vi "Convert cxd file.vi"(8 "error in (no error)":errorcluster, 11 "TomoConversion in":refnum<class "TomoConversion.lvclass">) -> (0 "error out":errorcluster, 3 "TomoConversion out":refnum<class "TomoConversion.lvclass">)   [LabVIEW 2012, in "TomoConversion.lvclass"]
uses:
  TomoConversion.lvclass
  TomoConversion.lvclass/TomoConversion.ctl
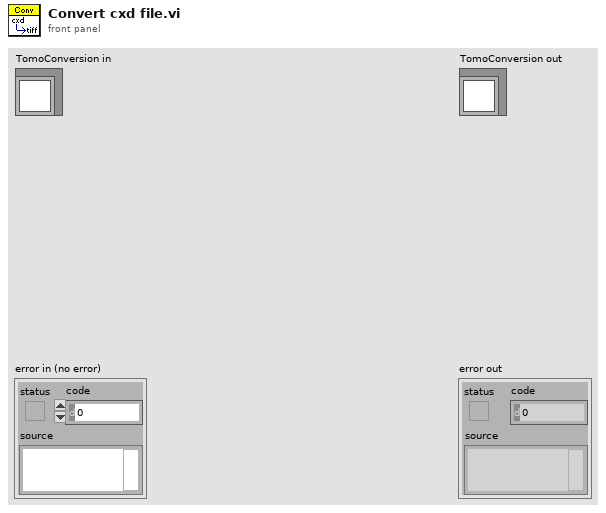
[diagram p1: front panel]
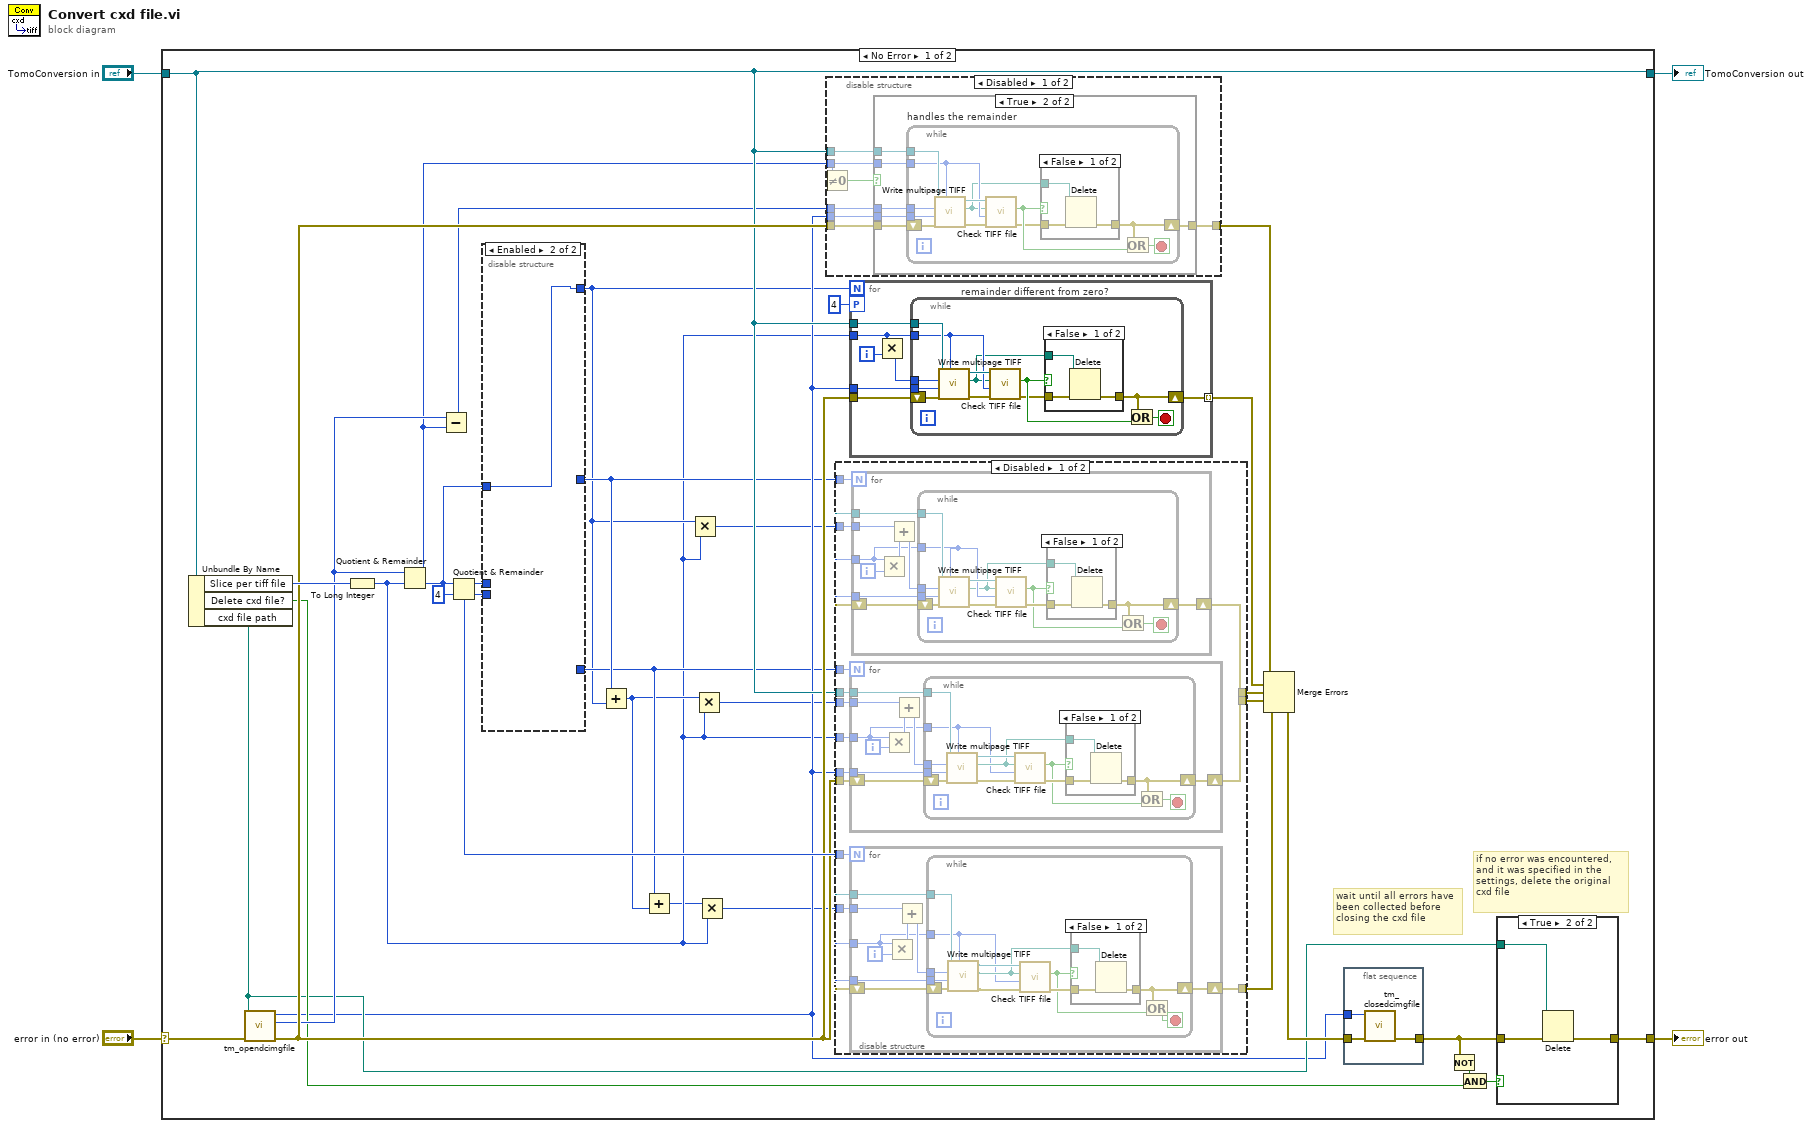
[diagram p0: block diagram]
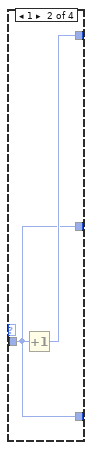
[diagram p3: hidden frame]
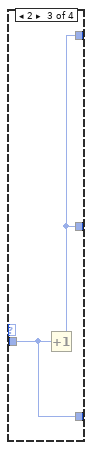
[diagram p4: hidden frame]
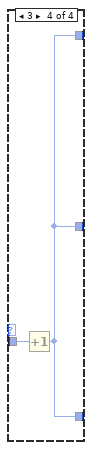
[diagram p5: hidden frame]
diagram:
  n1 = case shown="No Error" "error in (no error)" {
    selector: "error in (no error)" -> [w31 w201]
    tunnel: [w20 w201] -> w3
    tunnel: [w29 w200] -> w1
    tunnel: "TomoConversion in" -> [w29 w200]
    frame No Error {
      # "wait until all errors have\nbeen collected before\nclosing the cxd file"
      # "if no error was encountered, \nand it was specified in the \nsettings, delete the original\ncxd file"
      n2 = Unbundle By Name(w29) -> ("Slice per tiff file"=w38:u32, "Delete cxd file?"=w23:bool, "cxd file path"=w19:path)
      n3 = call <userlib>:"tm_opendcimgfile.vi"("error in (no error)"=w31, "Path"=w19) -> ("error out"=w30:errorcluster, "Total Frames"=w28:i32, "File Handle"=w17:u32)  [unwired: 7 in]
      n4 = To Long Integer(number=w38) -> (32bit integer=w9:i32)
      n5 = Quotient & Remainder(x=w28, y=w9) -> (x-y*floor(x/y)=w18:i32, floor(x/y)=w6:i32)
      n6 = Subtract(x=w28, y=w18) -> (x-y=w27:i32)
      n7 = Quotient & Remainder(x=w6, y=4) -> (x-y*floor(x/y)=w16:i32, floor(x/y)=w36:i32)
      n8 = disable-structure shown="Enabled" {
        disable-tunnel: w36 -> [w43 _]
        disable-tunnel: w16 -> [w42 _]
        disable-tunnel: [w41 _] -> w15
        disable-tunnel: [w40 _] -> w14
        disable-tunnel: [w39 w51] -> w13
        disable-tunnel: w6 -> [_ w51]
        frame Disabled {
          n9 = case shown="0, Default" w42 {
            tunnel: w43 -> [w44 w45 w48 w50]
            tunnel: [w44 w46 w47 w49] -> w39
            tunnel: [w44 w45 w47 w49] -> w41
            tunnel: [w44 w45 w48 w49] -> w40
            frame 0, Default {
            }
            frame 1 {
              n10 = Increment(x=w45) -> (x+1=w46:i32)
            }
            frame 2 {
              n11 = Increment(x=w48) -> (x+1=w47:i32)
            }
            frame 3 {
              n12 = Increment(x=w50) -> (x+1=w49:i32)
            }
          }
        }
        frame Enabled {
        }
      }
      n13 = Add(x=w15, y=w13) -> (x+y=w11:i32)
      n14 = Add(x=w14, y=w11) -> (x+y=w8:i32)
      n15 = Multiply(x=w13, y=w9) -> (x*y=w12:i32)
      n16 = Multiply(x=w11, y=w9) -> (x*y=w10:i32)
      n17 = Multiply(x=w8, y=w9) -> (x*y=w7:i32)
      n18 = disable-structure shown="Disabled" {
        disable-tunnel: w30 -> [w146 _]
        disable-tunnel: w29 -> [w145 _]
        disable-tunnel: w27 -> [w144 _]
        disable-tunnel: [w143 _] -> w26
        disable-tunnel: w18 -> [w141 _]
        disable-tunnel: w17 -> [w140 _]
        frame Disabled {
          n19 = Not Equal To 0?(x=w141) -> (x != 0?=w142:bool)
          n20 = case "remainder different from zero?" shown="True" w142 {
            tunnel: w146 -> [w147 w153]
            tunnel: w145 -> [_ w152]
            tunnel: w141 -> [_ w151]
            tunnel: w144 -> [_ w150]
            tunnel: [w147 w149] -> w143
            tunnel: w140 -> [_ w148]
            frame False {
            }
            frame True {
              n21 = while "handles the remainder" {
                tunnel: w148 -> [w164]
                tunnel: w152 -> [w163]
                tunnel: w151 -> [w160]
                shift-right: [w155] -> w149
                shift-left: w153 -> [w165]
                tunnel: w150 -> [w154]
                stop <- w159 stop-if-true
                n22 = call-dynamic "Write multipage TIFF.vi"("number of TIFF slices"=w160, "error in (no error)"=w165, "cxd file handle"=w164, "offset"=w154, "TomoConversion in"=w163) -> ("error out"=w162:errorcluster, "TIFF file path"=w156:path, "TomoConversion out"=w161:refnum<class "TomoConversion.lvclass">)  [unwired: 4 in]
                n23 = call-dynamic "Check TIFF file.vi"("error in (no error)"=w162, "Expected TIFF slices"=w160, "TIFF File path"=w156, "TomoConversion in"=w161) -> ("error out"=w157:errorcluster, "is fine?"=w158:bool)  [unwired: 5 in, 1 out]
                n24 = case shown="False" w158 {
                  tunnel: w157 -> [w168 w169]
                  tunnel: w156 -> [w167 _]
                  tunnel: [w166 w169] -> w155
                  frame False {
                    n25 = Delete(path (use dialog)=w167, error in=w168) -> (error out=w166:errorcluster)  [unwired: 3 in, 2 out]
                  }
                  frame True {
                  }
                }
                n26 = Or(x=w155, y=w158) -> (x .or. y?=w159:bool)
              }
            }
          }
        }
        frame Enabled {
        }
      }
      n27 = disable-structure shown="Disabled" {
        disable-tunnel: w36 -> [w64 _]
        disable-tunnel: [w63 _] -> w34
        disable-tunnel: [w62 _] -> w33
        disable-tunnel: [w61 _] -> w32
        disable-tunnel: w30 -> [w60 _]
        disable-tunnel: w29 -> [w59 _]
        disable-tunnel: w17 -> [w58 _]
        disable-tunnel: w15 -> [w57 _]
        disable-tunnel: w14 -> [w56 _]
        disable-tunnel: w12 -> [w55 _]
        disable-tunnel: w10 -> [w54 _]
        disable-tunnel: w9 -> [w53 _]
        disable-tunnel: w7 -> [w52 _]
        frame Disabled {
          n28 = for {
            N: w56 -> [_]
            tunnel: w53 -> [w66]
            tunnel: w59 -> [w67]
            shift-right: [w70] -> w62
            shift-left: w60 -> [w71]
            tunnel: w58 -> [w69]
            tunnel: w54 -> [w65]
            i -> [w73]
            n29 = Multiply(x=w66, y=w73) -> (x*y=w72:i32)
            n30 = Add(x=w65, y=w72) -> (x+y=w68:i32)
            n31 = while {
              tunnel: w69 -> [w84]
              tunnel: w68 -> [w83]
              tunnel: w67 -> [w82]
              tunnel: w66 -> [w75]
              shift-right: [w78] -> w70
              shift-left: w71 -> [w85]
              stop <- w74 stop-if-true
              n32 = call-dynamic "Write multipage TIFF.vi"("number of TIFF slices"=w75, "error in (no error)"=w85, "cxd file handle"=w84, "offset"=w83, "TomoConversion in"=w82) -> ("error out"=w79:errorcluster, "TIFF file path"=w76:path, "TomoConversion out"=w77:refnum<class "TomoConversion.lvclass">)  [unwired: 4 in]
              n33 = call-dynamic "Check TIFF file.vi"("error in (no error)"=w79, "Expected TIFF slices"=w75, "TIFF File path"=w76, "TomoConversion in"=w77) -> ("error out"=w81:errorcluster, "is fine?"=w80:bool)  [unwired: 5 in, 1 out]
              n34 = case shown="False" w80 {
                tunnel: w81 -> [w88 w89]
                tunnel: w76 -> [w87 _]
                tunnel: [w86 w89] -> w78
                frame False {
                  n35 = Delete(path (use dialog)=w87, error in=w88) -> (error out=w86:errorcluster)  [unwired: 3 in, 2 out]
                }
                frame True {
                }
              }
              n36 = Or(x=w78, y=w80) -> (x .or. y?=w74:bool)
            }
          }
          n37 = for {
            N: w64 -> [_]
            tunnel: w53 -> [w116]
            tunnel: w59 -> [w117]
            shift-right: [w120] -> w61
            shift-left: w60 -> [w121]
            tunnel: w58 -> [w119]
            tunnel: w52 -> [w115]
            i -> [w123]
            n38 = Multiply(x=w116, y=w123) -> (x*y=w122:i32)
            n39 = Add(x=w115, y=w122) -> (x+y=w118:i32)
            n40 = while {
              tunnel: w119 -> [w134]
              tunnel: w118 -> [w133]
              tunnel: w117 -> [w132]
              tunnel: w116 -> [w124]
              shift-right: [w128] -> w120
              shift-left: w121 -> [w135]
              stop <- w129 stop-if-true
              n41 = call-dynamic "Write multipage TIFF.vi"("number of TIFF slices"=w124, "error in (no error)"=w135, "cxd file handle"=w134, "offset"=w133, "TomoConversion in"=w132) -> ("error out"=w127:errorcluster, "TIFF file path"=w125:path, "TomoConversion out"=w126:refnum<class "TomoConversion.lvclass">)  [unwired: 4 in]
              n42 = call-dynamic "Check TIFF file.vi"("error in (no error)"=w127, "Expected TIFF slices"=w124, "TIFF File path"=w125, "TomoConversion in"=w126) -> ("error out"=w131:errorcluster, "is fine?"=w130:bool)  [unwired: 5 in, 1 out]
              n43 = case shown="False" w130 {
                tunnel: w131 -> [w138 w139]
                tunnel: w125 -> [w137 _]
                tunnel: [w136 w139] -> w128
                frame False {
                  n44 = Delete(path (use dialog)=w137, error in=w138) -> (error out=w136:errorcluster)  [unwired: 3 in, 2 out]
                }
                frame True {
                }
              }
              n45 = Or(x=w128, y=w130) -> (x .or. y?=w129:bool)
            }
          }
          n46 = for {
            N: w57 -> [_]
            tunnel: w53 -> [w91]
            tunnel: w59 -> [w92]
            shift-right: [w96] -> w63
            shift-left: w60 -> [w95]
            tunnel: w58 -> [w94]
            tunnel: w55 -> [w90]
            i -> [w98]
            n47 = Multiply(x=w91, y=w98) -> (x*y=w97:i32)
            n48 = Add(x=w90, y=w97) -> (x+y=w93:i32)
            n49 = while {
              tunnel: w94 -> [w109]
              tunnel: w93 -> [w108]
              tunnel: w92 -> [w107]
              tunnel: w91 -> [w104]
              shift-right: [w100] -> w96
              shift-left: w95 -> [w110]
              stop <- w101 stop-if-true
              n50 = call-dynamic "Write multipage TIFF.vi"("number of TIFF slices"=w104, "error in (no error)"=w110, "cxd file handle"=w109, "offset"=w108, "TomoConversion in"=w107) -> ("error out"=w105:errorcluster, "TIFF file path"=w102:path, "TomoConversion out"=w106:refnum<class "TomoConversion.lvclass">)  [unwired: 4 in]
              n51 = call-dynamic "Check TIFF file.vi"("error in (no error)"=w105, "Expected TIFF slices"=w104, "TIFF File path"=w102, "TomoConversion in"=w106) -> ("error out"=w103:errorcluster, "is fine?"=w99:bool)  [unwired: 5 in, 1 out]
              n52 = case shown="False" w99 {
                tunnel: w103 -> [w113 w114]
                tunnel: w102 -> [w112 _]
                tunnel: [w111 w114] -> w100
                frame False {
                  n53 = Delete(path (use dialog)=w112, error in=w113) -> (error out=w111:errorcluster)  [unwired: 3 in, 2 out]
                }
                frame True {
                }
              }
              n54 = Or(x=w100, y=w99) -> (x .or. y?=w101:bool)
            }
          }
        }
        frame Enabled {
        }
      }
      n55 = for {
        N: w13 -> [_]
        tunnel: w9 -> [w177]
        tunnel: w29 -> [w178]
        tunnel: w17 -> [w180]
        workers-P: 4 -> [_]
        tunnel: w30 -> [w181]
        tunnel: [w182] -> w35 mode=indexing
        i -> [w183]
        n56 = Multiply(x=w177, y=w183) -> (x*y=w179:i32)
        n57 = while {
          tunnel: w180 -> [w194]
          tunnel: w179 -> [w193]
          tunnel: w178 -> [w192]
          tunnel: w177 -> [w189]
          shift-right: [w185] -> w182
          shift-left: w181 -> [w195]
          stop <- w188 stop-if-true
          n58 = call-dynamic "Write multipage TIFF.vi"("number of TIFF slices"=w189, "error in (no error)"=w195, "cxd file handle"=w194, "offset"=w193, "TomoConversion in"=w192) -> ("error out"=w191:errorcluster, "TIFF file path"=w186:path, "TomoConversion out"=w190:refnum<class "TomoConversion.lvclass">)  [unwired: 4 in]
          n59 = call-dynamic "Check TIFF file.vi"("error in (no error)"=w191, "Expected TIFF slices"=w189, "TIFF File path"=w186, "TomoConversion in"=w190) -> ("error out"=w184:errorcluster, "is fine?"=w187:bool)  [unwired: 5 in, 1 out]
          n60 = case shown="False" w187 {
            tunnel: w184 -> [w198 w199]
            tunnel: w186 -> [w197 _]
            tunnel: [w196 w199] -> w185
            frame False {
              n61 = Delete(path (use dialog)=w197, error in=w198) -> (error out=w196:errorcluster)  [unwired: 3 in, 2 out]
            }
            frame True {
            }
          }
          n62 = Or(x=w185, y=w187) -> (x .or. y?=w188:bool)
        }
      }
      n63 = Merge Errors(w26, w35, w34, w33, w32) -> (w25:errorcluster)
      n64 = flat-sequence {
        tunnel: w25 -> [w172]
        tunnel: [w171] -> w21
        tunnel: w17 -> [w170]
        frame #0 {
          n65 = call <userlib>:"tm_closedcimgfile.vi"("error in (no error)"=w172, "File Handle"=w170) -> ("error out"=w171:errorcluster)  [unwired: 9 in]
        }
      }
      n66 = Not(x=w21) -> (.not. x?=w24:bool)
      n67 = And(x=w24, y=w23) -> (x .and. y?=w22:bool)
      n68 = case shown="True" w22 {
        tunnel: w21 -> [w173 w176]
        tunnel: [w173 w175] -> w20
        tunnel: w19 -> [_ w174]
        frame False {
        }
        frame True {
          n69 = Delete(path (use dialog)=w174, error in=w176) -> (error out=w175:errorcluster)  [unwired: 3 in, 2 out]
        }
      }
    }
    frame Error {
    }
  }
  "error out" <- w3
  "TomoConversion out" <- w1
